vi "Get Master-Slave Velocity Update Interval.vi"(4 "error in (no error)":errorcluster, 7 "VISA resource name":refnum<visa-resource-name>) -> (0 "error out":errorcluster, 2 "Interval (ms)":i32, 3 "VISA resource name out":refnum<visa-resource-name>)   [LabVIEW 2018, in "Newport ESP301.lvlib"]
doc: "the controller returns slave axis jog velocity update interval."
uses:
  Newport ESP301.lvlib
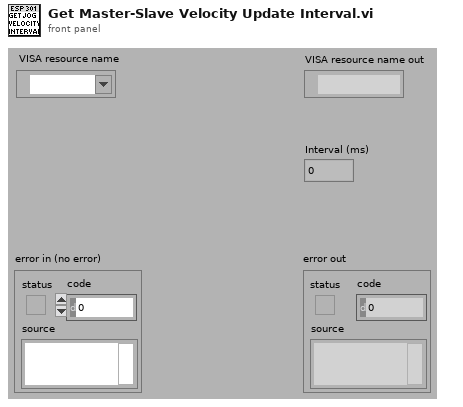
[diagram p1: front panel]
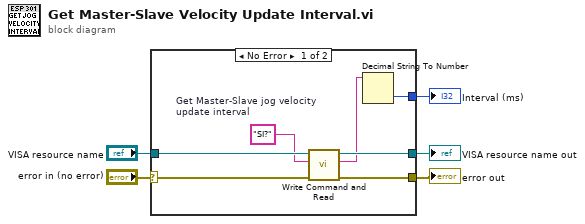
[diagram p0: block diagram]
diagram:
  n1 = case shown="No Error" "error in (no error)" {
    selector: "error in (no error)" -> [w11 w14]
    tunnel: [w8 w14] -> w5
    tunnel: "VISA resource name" -> [w12 w13]
    tunnel: [w10 w13] -> w4
    tunnel: [w9 _] -> w1
    frame No Error {
      w6 = "SI?"  # Get Master-Slave jog velocity  update interval
      n2 = call "Write Command and Read.vi"("error in (no error)"=w11, "Command"=w6, "VISA resource name"=w12) -> ("error out"=w8:errorcluster, "Returned string"=w7:string, "VISA resource name out"=w10:refnum<visa-resource-name>)  [unwired: 2 in, 2 out]
      n3 = Decimal String To Number(string=w7) -> (number=w9:i32)  [unwired: 1 in, 2 out]
    }
    frame Error {
    }
  }
  "error out" <- w5
  "VISA resource name out" <- w4
  "Interval (ms)" <- w1
